vi "PKG_IMC_Arc_Pos.vi"(0 "handle":u32, 1 "cy":i32, 2 "tgvel":dbl, 3 "wait":i32, 5 "endx":i32, 7 "endy":i32, 9 "cx":i32, 12 "dir":i32, 13 "endvel":dbl, 14 "fifo":i32) -> (4 "handle out":u32, 6 "function return":i32)   [LabVIEW 2011, in "IMC_Pkg4xxx.lvlib"]
doc: "PKG_IMC_Arc_Pos(IMC_HANDLE handle, long endx, long endy, long cx, long cy, int dir, double tgvel, double endvel, int wait, int fifo) ;"
uses:
  IMC_Pkg4xxx.lvlib
  IMC_Pkg4xxx.dll
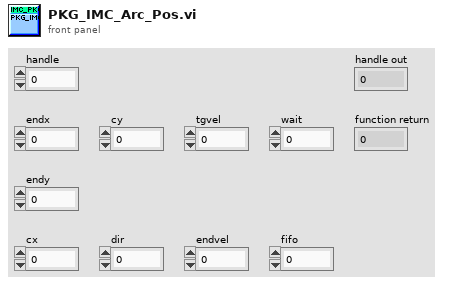
[diagram p1: front panel]
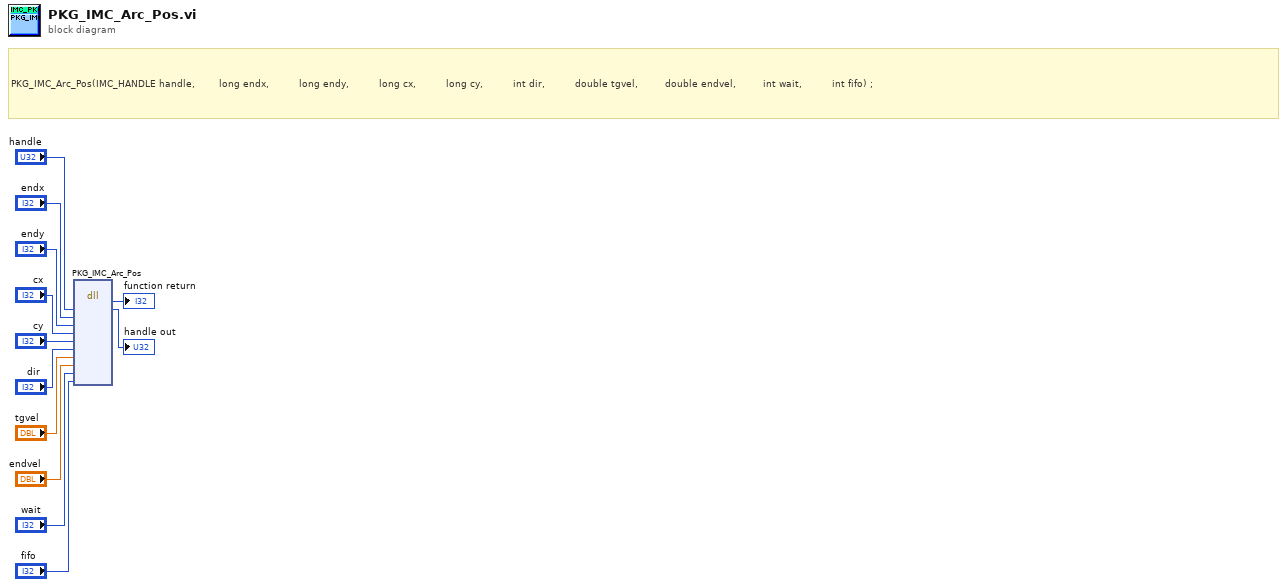
[diagram p0: block diagram]
diagram:
  # "PKG_IMC_Arc_Pos(IMC_HANDLE handle, \t\t\t\t\t\t\tlong endx, \t\t\t\t\t\t\t\t\tlong endy, \t\t\t\t\t\t\t\t\tlong cx, \t\t\t\t\t\t\t\t\tlong cy, \t\t\t\t\t\t\t\t\tint dir, \t\t\t\t\t\t\t\t\tdouble tgvel, \t\t\t\t\t\t\t\tdouble endvel, \t\t\t\t\t\t\t\tint wait, \t\t\t\t\t\t\t\t\tint fifo) ;"
  n1 = dll-call lib="PTH1`abs F光盘刻录\niMC MotionIMCNet_V4.0IMCAppincLabviewIMC_PKG4xxx\nIMC_Pkg4xxx.*" fn="PKG_IMC_Arc_Pos"("handle"="handle", "endx"="endx", "endy"="endy", "cx"="cx", "cy"="cy", "dir"="dir", "tgvel"="tgvel", "endvel"="endvel", "wait"="wait", "fifo"="fifo") -> ("返回类型"=→"function return":i32, "handle"=→"handle out":u32)  [unwired: 12 in, 2 out]
